vi "Transform.vi"(8 "error in (no error)":errorcluster, 11 "XRay Table in":refnum<class "XRay Table.lvclass">=refnum) -> (0 "error out":errorcluster, 3 "XRay Table out":refnum<class "XRay Table.lvclass">)   [LabVIEW 2026, in "XRay Table.lvclass"]
uses:
  XRay Table.lvclass
  XRay Table.lvclass/XRay Table.ctl
  <vilib>/picture/3D Picture Control/NI_3D Picture Control.lvlib
panel:
  in  "Translation 4":cluster{"X":sgl, "Y":sgl, "Z":sgl}={"X"=3.0, "Y"=-0.5, "Z"=0.0}
  in  "Translation 3":cluster{"X":sgl, "Y":sgl, "Z":sgl}={"X"=5.0, "Y"=7.0, "Z"=0.5}
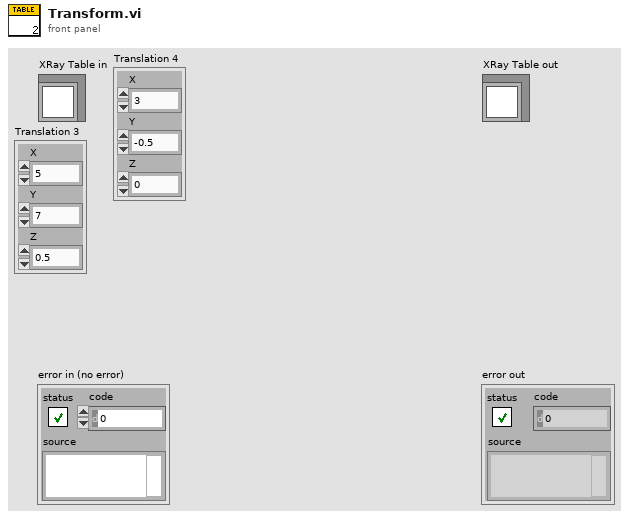
[diagram p1: front panel]
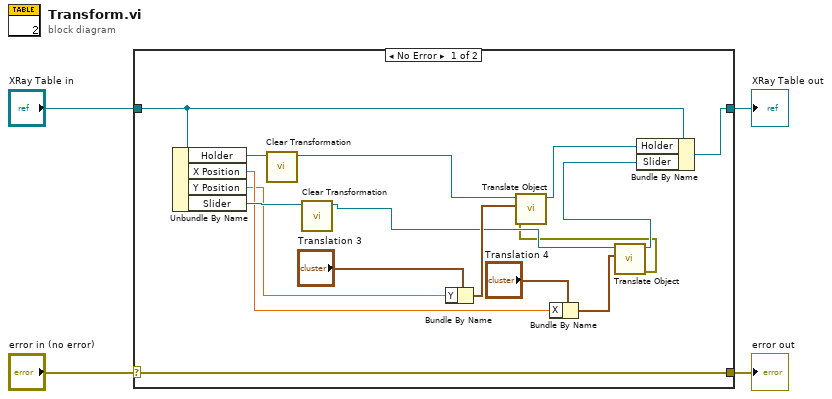
[diagram p0: block diagram]
diagram:
  n1 = case shown="No Error" "error in (no error)" {
    selector: "error in (no error)" -> [w20 w22]
    tunnel: [w20 w22] -> w3
    tunnel: [w15 w21] -> w1
    tunnel: "XRay Table in" -> [w17 w21]
    frame No Error {
      n2 = Unbundle By Name(w17) -> ("Holder"=w19:refnum<vi>, "X Position"=w8:dbl, "Y Position"=w6:dbl, "Slider"=w10:refnum<vi>)
      n3 = call <vilib>:"Clear Transformation.vi"("Object Refnum In"=w19) -> ("Object Refnum Out"=w18:refnum<vi>)  [unwired: 1 in, 9 out]
      n4 = call <vilib>:"Clear Transformation.vi"("Object Refnum In"=w10) -> ("Object Refnum Out"=w9:refnum<vi>)  [unwired: 1 in, 9 out]
      n5 = Bundle By Name(cluster="Translation 3", "Y"=w6) -> (w13:cluster{"X":sgl, "Y":sgl, "Z":sgl})
      n6 = Bundle By Name(cluster="Translation 4", "X"=w8) -> (w12:cluster{"X":sgl, "Y":sgl, "Z":sgl})
      n7 = call <vilib>:"Translate Object.vi"("Translation"=w12, "Scene.Object In"=w9) -> ("error out"=w7:errorcluster, "Scene.Object Out"=w11:refnum<vi>)  [unwired: 8 in]
      n8 = call <vilib>:"Translate Object.vi"("error in (no error)"=w7, "Translation"=w13, "Scene.Object In"=w18) -> ("Scene.Object Out"=w16:refnum<vi>)  [unwired: 7 in, 1 out]
      n9 = Bundle By Name(cluster=w17, "Holder"=w16, "Slider"=w11) -> (w15:refnum<class "XRay Table.lvclass">)
    }
    frame Error {
    }
  }
  "error out" <- w3
  "XRay Table out" <- w1
